vi "Build New AIM MIL-STD-1553 Custom Device.vi"() -> ()   [LabVIEW 2020]
uses:
  <vilib>/addons/VeriStand Custom Device Scripting APIs/AIM MIL-STD-1553/Shared/AIM Hardware Parameters.ctl
  <vilib>/addons/VeriStand Custom Device Scripting APIs/AIM MIL-STD-1553/Shared/Initialization Method.ctl
  <vilib>/addons/VeriStand Custom Device Scripting APIs/AIM MIL-STD-1553/Shared/Bus Selection.ctl
  <vilib>/addons/VeriStand Custom Device Scripting APIs/AIM MIL-STD-1553/Shared/Coupling Mode.ctl
  <vilib>/addons/VeriStand Custom Device Scripting APIs/AIM MIL-STD-1553/Shared/BIU Configuration.ctl
  <vilib>/addons/VeriStand Custom Device Scripting APIs/AIM MIL-STD-1553/Shared/Address.ctl
  <vilib>/addons/VeriStand Custom Device Scripting APIs/AIM MIL-STD-1553/Shared/Major Frame Definition.ctl
  <vilib>/addons/VeriStand Custom Device Scripting APIs/AIM MIL-STD-1553/Shared/Minor Frame Definition.ctl
  <vilib>/addons/VeriStand Custom Device Scripting APIs/AIM MIL-STD-1553/Shared/Acyclic Frame Definition.ctl
  <vilib>/addons/VeriStand Custom Device Scripting APIs/AIM MIL-STD-1553/Shared/Message Definition.ctl
  <vilib>/addons/VeriStand Custom Device Scripting APIs/AIM MIL-STD-1553/Shared/Message Type.ctl
  <vilib>/addons/VeriStand Custom Device Scripting APIs/AIM MIL-STD-1553/Shared/Terminal Endpoint.ctl
  <vilib>/addons/VeriStand Custom Device Scripting APIs/AIM MIL-STD-1553/Shared/Parameter Definition.ctl
  AIM MIL-STD-1553 Scripting Example Support.lvlib
  <vilib>/addons/VeriStand Custom Device Scripting APIs/AIM MIL-STD-1553/Scripting/AIM MIL-STD-1553 Scripting.lvlib
  NationalInstruments.VeriStand.SystemDefinitionAPI
panel:
  in  "Example Documentation":string="Overview: Demonstrates using the AIM MIL-STD-1553 scripting API to add and configure a new custom device from configuration data. \n\nInstructions:\n1. Specify the PXI Slot Number and Core Number for your AIM MIL-STD-1553 hardware.\n2. (VeriStand) Optionally, to perform avionics bus communications with AIM MIL-STD-1553 hardware you may:\n   a. Open the AIM MIL-STD-1553 System Definition in VeriStand.\n   b. Configure the PXI Linux RT Target.\n   c. Deploy the scripted system definition."
  in  "BIU Number":i32=1
  in  "PXI Slot Number":i32=2
  in  "Base System Definition File":path=path "Support/Base.nivssdf"
  in  "Output System Definition File":path=path "Support/Scripted Configuration AIM MIL-STD-1553.nivssdf"
  out "AIM MIL-STD-1553 System Definition":path
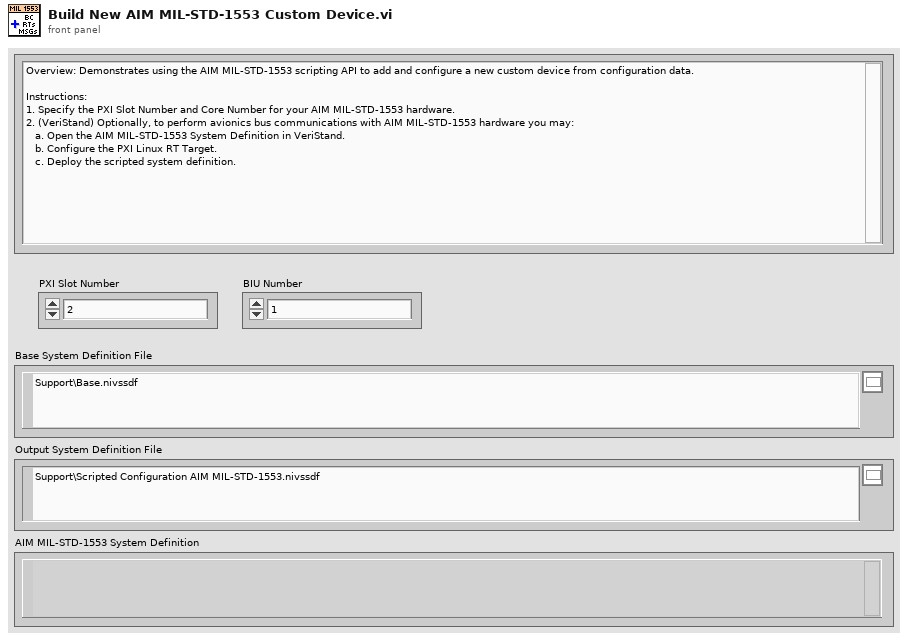
[diagram p1: front panel]
types:
  T1 = typedef "BIU Configuration.ctl" = cluster{"HW channel":u16, "terminal addresses":T2[], "terminal names":string[], "major frames":T3[], "minor frames":T4[], "acyclic frames":T5[], "messages":T6[]}
  T2 = typedef "Address.ctl" = u16
  T3 = typedef "Major Frame Definition.ctl" = cluster{"name":string, "minor frames":string[]}
  T4 = typedef "Minor Frame Definition.ctl" = cluster{"name":string, "messages":string[]}
  T5 = typedef "Acyclic Frame Definition.ctl" = cluster{"name":string, "messages":string[]}
  T6 = typedef "Message Definition.ctl" = cluster{"name":string, "message type":T7, "endpoint Tx":T8, "endpoint Rx":T8, "create timestamp channel":bool, "mode code":u16, "number of words":u16, "parameters":cluster{"name":string, "default value":dbl, "unit":string, "parameter definition":T9}[]}
  T7 = typedef "Message Type.ctl" = string
  T8 = typedef "Terminal Endpoint.ctl" = cluster{"terminal address":T2, "subaddress":T2}
  T9 = typedef "Parameter Definition.ctl" = cluster{"start index":i32, "size (bits)":i32, "encoding":enum16{"BNR", "BCD", "Discrete"}, "signed":bool, "multiplier":dbl, "offset":dbl}
  T10 = typedef "AIM Hardware Parameters.ctl" = cluster{"initialization method":T11, "card number":i32, "pxi slot number":i32, "biu number":i32, "bus selection":T12, "coupling mode":T13}
  T11 = typedef "Initialization Method.ctl" = enum16{"PXI Slot Number", "Card Number"}
  T12 = typedef "Bus Selection.ctl" = enum16{"Both", "Primary", "Secondary"}
  T13 = typedef "Coupling Mode.ctl" = enum16{"Isolated Onboard Termination", "Transformer Coupled", "Direct Coupled", "External with Onboard Termination", "Onboard Digital Wrap-around"}
  T14 = typedef "Custom Device API.lvlib/Custom Device Item Ref.ctl" = u64
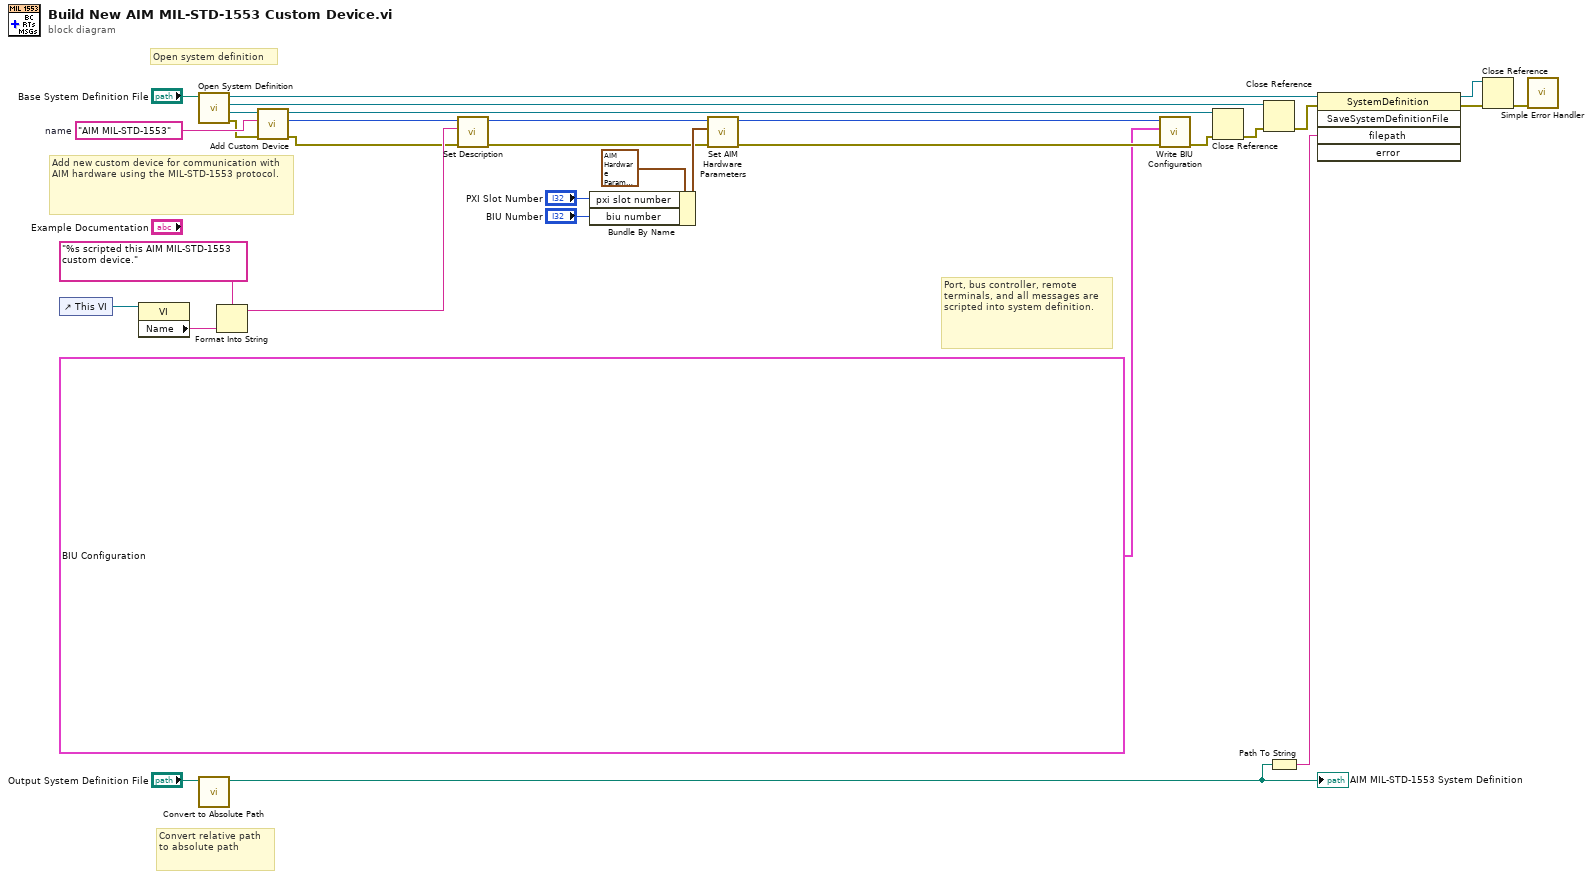
[diagram p0: block diagram]
diagram:
  w21 = "AIM MIL-STD-1553"  # name
  # "Port, bus controller, remote terminals, and all messages are scripted into system definition."
  # "Add new custom device for communication with AIM hardware using the MIL-STD-1553 protocol."
  # "Convert relative path to absolute path"
  # "Open system definition"
  # "8."
  n1 = control-ref of="This VI"() -> (w15:refnum<vi>)
  n2 = property class="VI"(reference=w15) -> ("Name"=w14:string)  [unwired: 1 in, 2 out]
  n3 = call "Open System Definition.vi"("system definition file"="Base System Definition File") -> ("error out"=w17:errorcluster, "target"=w23:refnum<k24>, "root"=w19:refnum<k24>, "system definition"=w18:refnum<k24>)  [unwired: 7 in]
  n4 = call "Convert to Absolute Path.vi"("system definition file"="Output System Definition File") -> ("absolute path"=w22:path)  [unwired: 10 in]
  "AIM MIL-STD-1553 System Definition" <- w22
  n5 = Format Into String(format string="%s scripted this AIM MIL-STD-1553 custom device." ("description"), w14) -> (resulting string=w13:string)  [unwired: 2 in, 1 out]
  n6 = call <vilib>:"Add Custom Device.vi"("error in"=w17, "custom device name"=w21, "target"=w23) -> ("error out"=w11:errorcluster, "custom device"=w12:T14, "target out"=w20:refnum<k24>)  [unwired: 6 in]
  n7 = call <vilib>:"Set Description.vi"("error in"=w11, "description"=w13, "custom device"=w12) -> ("error out"=w7:errorcluster, "custom device out"=w10:T14)  [unwired: 7 in]
  n8 = Bundle By Name(cluster=T10 {"initialization method"=enum."PXI Slot Number", "card number"=0, "pxi slot number"=2, "biu number"=0, "bus selection"=enum."Both", "coupling mode"=enum."Isolated Onboard Termination"} ("device parameters"), "pxi slot number"="PXI Slot Number", "biu number"="BIU Number") -> (w8:T10)
  n9 = call <vilib>:"Set AIM Hardware Parameters.vi"("error in"=w7, "aim hardware parameters"=w8, "custom device"=w10) -> ("error out"=w4:errorcluster, "custom device out"=w3:T14)  [unwired: 7 in]
  n10 = call <vilib>:"Write BIU Configuration.vi"("error in"=w4, "biu configuration"=T1 {"HW channel"=0, "terminal addresses"=[0, 1, 2, 15, 30], "terminal names"=["Bus Controller", "Remote Terminal 01", "Remote Terminal 02", "Remote Terminal 15", "Remote Terminal 30"], "major frames"=[{"name"="MajorCycle", "minor frames"=["Cycle50Hz", "Cycle25Hz"]}], "minor frames"=[{"name"="Cycle50Hz", "messages"=["BC to RT 1.1", "BC to RT 2.1", "RT 1.4 to BC", "RT 2.3 to RT 30.2", "RT 30.28 to RT 2.4", "MC 16"]}, {"name"="Cycle25Hz", "messages"=["BC to RT 1.2", "RT 2.2 to BC", "RT 30.1 to BC", "RT 15.22 to RT 30.22", "MC 01", "MC 17"]}], "acyclic frames"=[{"name"="acyclicFrame 1", "messages"=["BC to RT 1.3"]}, {"name"="acyclicFrame 2", "messages"=["RT 1.6 to RT 2.7", "RT 1.5 to BC"]}], "messages"=[{"name"="BC to RT 1.1", "message type"="BC to RT", "endpoint Tx"={"terminal address"=0, "subaddress"=0}, "endpoint Rx"={"terminal address"=1, "subaddress"=1}, "create timestamp channel"=TRUE, "mode code"=0, "number of words"=2, "parameters"=[{"name"="Word 00", "default value"=0.0, "unit"="", "parameter definition"={"start index"=0, "size (bits)"=16, "encoding"=enum."BNR", "signed"=FALSE, "multiplier"=1.0, "offset"=0.0}}, {"name"="Word 01", "default value"=0.0, "unit"="", "parameter definition"={"start index"=16, "size (bits)"=16, "encoding"=enum."BNR", "signed"=FALSE, "multiplier"=1.0, "offset"=0.0}}]}, {"name"="BC to RT 1.2", "message type"="BC to RT", "endpoint Tx"={"terminal address"=0, "subaddress"=0}, "endpoint Rx"={"terminal address"=1, "subaddress"=2}, "create timestamp channel"=FALSE, "mode code"=0, "number of words"=1, "parameters"=[{"name"="Parameter 1.2.1", "default value"=1.0, "unit"="", "parameter definition"={"start index"=0, "size (bits)"=8, "encoding"=enum."BNR", "signed"=FALSE, "multiplier"=1.0, "offset"=0.0}}, {"name"="Parameter 1.2.2", "default value"=2.0, "unit"="", "parameter definition"={"start index"=8, "size (bits)"=8, "encoding"=enum."BNR", "signed"=FALSE, "multiplier"=1.0, "offset"=0.0}}]}, {"name"="BC to RT 1.3", "message type"="BC to RT", "endpoint Tx"={"terminal address"=0, "subaddress"=0}, "endpoint Rx"={"terminal address"=1, "subaddress"=3}, "create timestamp channel"=FALSE, "mode code"=0, "number of words"=3, "parameters"=[{"name"="Word 00", "default value"=0.0, "unit"="", "parameter definition"={"start index"=0, "size (bits)"=16, "encoding"=enum."BNR", "signed"=FALSE, "multiplier"=1.0, "offset"=0.0}}, {"name"="Word 01", "default value"=0.0, "unit"="", "parameter definition"={"start index"=16, "size (bits)"=16, "encoding"=enum."BNR", "signed"=FALSE, "multiplier"=1.0, "offset"=0.0}}, {"name"="Word 02", "default value"=0.0, "unit"="", "parameter definition"={"start index"=32, "size (bits)"=16, "encoding"=enum."BNR", "signed"=FALSE, "multiplier"=1.0, "offset"=0.0}}]}, {"name"="BC to RT 2.1", "message type"="BC to RT", "endpoint Tx"={"terminal address"=0, "subaddress"=0}, "endpoint Rx"={"terminal address"=2, "subaddress"=1}, "create timestamp channel"=FALSE, "mode code"=0, "number of words"=3, "parameters"=[{"name"="Word 00", "default value"=0.0, "unit"="", "parameter definition"={"start index"=0, "size (bits)"=16, "encoding"=enum."BNR", "signed"=FALSE, "multiplier"=1.0, "offset"=0.0}}, {"name"="Word 01", "default value"=0.0, "unit"="", "parameter definition"={"start index"=16, "size (bits)"=16, "encoding"=enum."BNR", "signed"=FALSE, "multiplier"=1.0, "offset"=0.0}}, {"name"="Word 02", "default value"=0.0, "unit"="", "parameter definition"={"start index"=32, "size (bits)"=16, "encoding"=enum."BNR", "signed"=FALSE, "multiplier"=1.0, "offset"=0.0}}]}, {"name"="MC 01", "message type"="MC", "endpoint Tx"={"terminal address"=0, "subaddress"=0}, "endpoint Rx"={"terminal address"=31, "subaddress"=31}, "create timestamp channel"=FALSE, "mode code"=1, "number of words"=0, "parameters"=[]}, {"name"="MC 16", "message type"="MC", "endpoint Tx"={"terminal address"=1, "subaddress"=31}, "endpoint Rx"={"terminal address"=0, "subaddress"=0}, "create timestamp channel"=FALSE, "mode code"=16, "number of words"=1, "parameters"=[{"name"="Word 00", "default value"=0.0, "unit"="", "parameter definition"={"start index"=0, "size (bits)"=16, "encoding"=enum."BNR", "signed"=FALSE, "multiplier"=1.0, "offset"=0.0}}]}, {"name"="MC 17", "message type"="MC", "endpoint Tx"={"terminal address"=0, "subaddress"=0}, "endpoint Rx"={"terminal address"=1, "subaddress"=31}, "create timestamp channel"=FALSE, "mode code"=17, "number of words"=1, "parameters"=[{"name"="Word 00", "default value"=0.0, "unit"="", "parameter definition"={"start index"=0, "size (bits)"=16, "encoding"=enum."BNR", "signed"=FALSE, "multiplier"=1.0, "offset"=0.0}}]}, {"name"="RT 1.4 to BC", "message type"="RT to BC", "endpoint Tx"={"terminal address"=1, "subaddress"=4}, "endpoint Rx"={"terminal address"=0, "subaddress"=0}, "create timestamp channel"=FALSE, "mode code"=0, "number of words"=3, "parameters"=[{"name"="Word 00", "default value"=0.0, "unit"="", "parameter definition"={"start index"=0, "size (bits)"=16, "encoding"=enum."BNR", "signed"=FALSE, "multiplier"=1.0, "offset"=0.0}}, {"name"="Word 01", "default value"=0.0, "unit"="", "parameter definition"={"start index"=16, "size (bits)"=16, "encoding"=enum."BNR", "signed"=FALSE, "multiplier"=1.0, "offset"=0.0}}, {"name"="Word 02", "default value"=0.0, "unit"="", "parameter definition"={"start index"=32, "size (bits)"=16, "encoding"=enum."BNR", "signed"=FALSE, "multiplier"=1.0, "offset"=0.0}}]}, {"name"="RT 1.5 to BC", "message type"="RT to BC", "endpoint Tx"={"terminal address"=1, "subaddress"=5}, "endpoint Rx"={"terminal address"=0, "subaddress"=0}, "create timestamp channel"=FALSE, "mode code"=0, "number of words"=3, "parameters"=[{"name"="Word 00", "default value"=0.0, "unit"="", "parameter definition"={"start index"=0, "size (bits)"=16, "encoding"=enum."BNR", "signed"=FALSE, "multiplier"=1.0, "offset"=0.0}}, {"name"="Word 01", "default value"=0.0, "unit"="", "parameter definition"={"start index"=16, "size (bits)"=16, "encoding"=enum."BNR", "signed"=FALSE, "multiplier"=1.0, "offset"=0.0}}, {"name"="Word 02", "default value"=0.0, "unit"="", "parameter definition"={"start index"=32, "size (bits)"=16, "encoding"=enum."BNR", "signed"=FALSE, "multiplier"=1.0, "offset"=0.0}}]}, {"name"="RT 1.6 to RT 2.7", "message type"="RT to RT", "endpoint Tx"={"terminal address"=1, "subaddress"=6}, "endpoint Rx"={"terminal address"=2, "subaddress"=7}, "create timestamp channel"=TRUE, "mode code"=0, "number of words"=3, "parameters"=[{"name"="Word 00", "default value"=0.0, "unit"="", "parameter definition"={"start index"=0, "size (bits)"=16, "encoding"=enum."BNR", "signed"=FALSE, "multiplier"=1.0, "offset"=0.0}}, {"name"="Word 01", "default value"=0.0, "unit"="", "parameter definition"={"start index"=16, "size (bits)"=16, "encoding"=enum."BNR", "signed"=FALSE, "multiplier"=1.0, "offset"=0.0}}, {"name"="Word 02", "default value"=0.0, "unit"="", "parameter definition"={"start index"=32, "size (bits)"=16, "encoding"=enum."BNR", "signed"=FALSE, "multiplier"=1.0, "offset"=0.0}}]}, {"name"="RT 15.22 to RT 30.22", "message type"="RT to RT", "endpoint Tx"={"terminal address"=15, "subaddress"=22}, "endpoint Rx"={"terminal address"=30, "subaddress"=22}, "create timestamp channel"=TRUE, "mode code"=0, "number of words"=3, "parameters"=[{"name"="Parameter 0", "default value"=0.0, "unit"="", "parameter definition"={"start index"=0, "size (bits)"=16, "encoding"=enum."BNR", "signed"=FALSE, "multiplier"=2.0, "offset"=0.0}}, {"name"="Parameter 1", "default value"=0.0, "unit"="", "parameter definition"={"start index"=16, "size (bits)"=16, "encoding"=enum."BNR", "signed"=FALSE, "multiplier"=1.0, "offset"=50.0}}, {"name"="Parameter 2", "default value"=0.0, "unit"="", "parameter definition"={"start index"=32, "size (bits)"=16, "encoding"=enum."BNR", "signed"=TRUE, "multiplier"=1.0, "offset"=0.0}}]}, {"name"="RT 2.2 to BC", "message type"="RT to BC", "endpoint Tx"={"terminal address"=2, "subaddress"=2}, "endpoint Rx"={"terminal address"=0, "subaddress"=0}, "create timestamp channel"=TRUE, "mode code"=0, "number of words"=8, "parameters"=[{"name"="Parameter 2.2.1", "default value"=21.0, "unit"="", "parameter definition"={"start index"=0, "size (bits)"=32, "encoding"=enum."BNR", "signed"=TRUE, "multiplier"=1.0, "offset"=0.0}}, {"name"="Parameter 2.2.2", "default value"=22.0, "unit"="", "parameter definition"={"start index"=32, "size (bits)"=32, "encoding"=enum."BNR", "signed"=FALSE, "multiplier"=1.0, "offset"=0.0}}, {"name"="Parameter 2.2.3", "default value"=23.0, "unit"="", "parameter definition"={"start index"=64, "size (bits)"=32, "encoding"=enum."BNR", "signed"=TRUE, "multiplier"=1.0, "offset"=0.0}}, {"name"="Parameter 2.2.4", "default value"=24.0, "unit"="", "parameter definition"={"start index"=96, "size (bits)"=32, "encoding"=enum."BNR", "signed"=FALSE, "multiplier"=1.0, "offset"=0.0}}]}, {"name"="RT 2.3 to RT 30.2", "message type"="RT to RT", "endpoint Tx"={"terminal address"=2, "subaddress"=3}, "endpoint Rx"={"terminal address"=30, "subaddress"=2}, "create timestamp channel"=TRUE, "mode code"=0, "number of words"=6, "parameters"=[{"name"="Word 00", "default value"=0.0, "unit"="", "parameter definition"={"start index"=0, "size (bits)"=16, "encoding"=enum."BNR", "signed"=FALSE, "multiplier"=1.0, "offset"=0.0}}, {"name"="Word 01", "default value"=0.0, "unit"="", "parameter definition"={"start index"=16, "size (bits)"=16, "encoding"=enum."BNR", "signed"=FALSE, "multiplier"=1.0, "offset"=0.0}}, {"name"="Word 02", "default value"=0.0, "unit"="", "parameter definition"={"start index"=32, "size (bits)"=16, "encoding"=enum."BNR", "signed"=FALSE, "multiplier"=1.0, "offset"=0.0}}, {"name"="Word 03", "default value"=0.0, "unit"="", "parameter definition"={"start index"=48, "size (bits)"=16, "encoding"=enum."BNR", "signed"=FALSE, "multiplier"=1.0, "offset"=0.0}}, {"name"="Word 04", "default value"=0.0, "unit"="", "parameter definition"={"start index"=64, "size (bits)"=16, "encoding"=enum."BNR", "signed"=FALSE, "multiplier"=1.0, "offset"=0.0}}, {"name"="Word 05", "default value"=0.0, "unit"="", "parameter definition"={"start index"=80, "size (bits)"=16, "encoding"=enum."BNR", "signed"=FALSE, "multiplier"=1.0, "offset"=0.0}}]}, {"name"="RT 30.1 to BC", "message type"="RT to BC", "endpoint Tx"={"terminal address"=30, "subaddress"=1}, "endpoint Rx"={"terminal address"=0, "subaddress"=0}, "create timestamp channel"=FALSE, "mode code"=0, "number of words"=2, "parameters"=[{"name"="Word 00", "default value"=0.0, "unit"="", "parameter definition"={"start index"=0, "size (bits)"=16, "encoding"=enum."BNR", "signed"=FALSE, "multiplier"=1.0, "offset"=0.0}}, {"name"="Word 01", "default value"=0.0, "unit"="", "parameter definition"={"start index"=16, "size (bits)"=16, "encoding"=enum."BNR", "signed"=FALSE, "multiplier"=1.0, "offset"=0.0}}]}, {"name"="RT 30.28 to RT 2.4", "message type"="RT to RT", "endpoint Tx"={"terminal address"=30, "subaddress"=28}, "endpoint Rx"={"terminal address"=2, "subaddress"=4}, "create timestamp channel"=FALSE, "mode code"=0, "number of words"=8, "parameters"=[{"name"="Parameter 30.28.1", "default value"=31.0, "unit"="", "parameter definition"={"start index"=0, "size (bits)"=32, "encoding"=enum."BNR", "signed"=TRUE, "multiplier"=1.0, "offset"=0.0}}, {"name"="Parameter 30.28.2", "default value"=32.0, "unit"="", "parameter definition"={"start index"=32, "size (bits)"=32, "encoding"=enum."BNR", "signed"=FALSE, "multiplier"=1.0, "offset"=0.0}}, {"name"="Parameter 30.28.3", "default value"=33.0, "unit"="", "parameter definition"={"start index"=64, "size (bits)"=32, "encoding"=enum."BNR", "signed"=TRUE, "multiplier"=1.0, "offset"=0.0}}, {"name"="Parameter 30.28.4", "default value"=34.0, "unit"="", "parameter definition"={"start index"=96, "size (bits)"=16, "encoding"=enum."BNR", "signed"=FALSE, "multiplier"=1.0, "offset"=0.0}}, {"name"="Parameter 30.28.5", "default value"=35.0, "unit"="", "parameter definition"={"start index"=112, "size (bits)"=16, "encoding"=enum."BNR", "signed"=FALSE, "multiplier"=1.0, "offset"=0.0}}]}]}, "custom device"=w3) -> ("error out"=w2:errorcluster)  [unwired: 7 in, 1 out]
  n11 = Close Reference(reference=w20, error in (no error)=w2) -> (error out=w24:errorcluster)
  n12 = Close Reference(reference=w19, error in (no error)=w24) -> (error out=w27:errorcluster)
  n13 = Path To String(path=w22) -> (string=w30:string)
  n14 = invoke class="SystemDefinition" method="SaveSystemDefinitionFile"(reference=w18, error in=w27, "filepath"=w30) -> (reference out=w28:refnum<k24>, error out=w29:errorcluster)  [unwired: 2 in, 3 out]
  n15 = Close Reference(reference=w28, error in (no error)=w29) -> (error out=w26:errorcluster)
  n16 = call <vilib>:"Simple Error Handler.vi"("error in (no error)"=w26) -> ()  [unwired: 1 in, 8 out]
